vi "Input.vi"(8 "error in (no error)":errorcluster, 11 "Pump Calibration Config in":T1={"Settings"={"Cycle Period"=500.0, "Ismatech"={"VISA resource name"="", "Simulated?"=TRUE, "Pump Number"=1.0, "Reverse?"=FALSE}, "Masterflex"={"VISA resource name"="", "Simulated?"=TRUE, "Pump Number"=1.0, "Reverse?"=FALSE}, "Bronkhorst M13 Settings"={"VISA resource name"="", "Simulated?"=TRUE, "Smoothing Steps"=1}, "PID 2 Parameters"={"Input Device"=enum."Default", "Output Device"=enum."Default"}, "Tacmina Settings"={"Analog DAQ Task"="", "Digital DAQ Task"=""}, "KNF SIMDOS Settings"={"VISA resource name"="", "Simulated?"=TRUE}, "VICI M50 Settings"={"VISA resource name"="", "Pump ID"="", "Pump Head Vol"=0.0, "Reverse?"=FALSE, "Simulated?"=TRUE}, "FLOM Settings"={"VISA resource name"="", "Simulated?"=TRUE, "Pump Number"=0.0}, "Calibration Limits"={"Minimum (ml/min)"=0.0, "Maximum (ml/min)"=0.0, "Steps"=0.0}, "SSI PR Settings"={"VISA resource name"="", "Simulated?"=FALSE}, "Ismatech 4308 Settings"={"VISA resource name"="", "Pump Number"=1, "Channel Number"=0, "Simulated?"=TRUE, "Reverse?"=FALSE}, "Bronkhorst M14 Settings"={"VISA resource name"="", "Simulated?"=FALSE, "Smoothing Steps"=1}}, "Flowmeter Output"=0.0, "Density"=0.0, "FL Temp"=0.0, "Speed %"=0.0, "File Refnum"=refnum, "Pump On?"=enum."Not Initialized"} {"Settings"."Bronkhorst M14 Settings"."Smoothing Steps" min=1 step=1; "Settings"."Ismatech 4308 Settings"."Channel Number" min=0 max=3; "Settings"."Ismatech 4308 Settings"."Pump Number" min=1; "Settings"."Bronkhorst M13 Settings"."Smoothing Steps" min=1 step=1; "Settings"."Masterflex"."Pump Number" min=1.0 max=20.0 step=1.0; "Settings"."Ismatech"."Pump Number" min=1.0 max=20.0 step=1.0}) -> (0 "error out":errorcluster, 3 "Pump Calibration Config Out":T1={"Settings"={"Cycle Period"=500.0, "Ismatech"={"VISA resource name"="", "Simulated?"=TRUE, "Pump Number"=1.0, "Reverse?"=FALSE}, "Masterflex"={"VISA resource name"="", "Simulated?"=TRUE, "Pump Number"=1.0, "Reverse?"=FALSE}, "Bronkhorst M13 Settings"={"VISA resource name"="", "Simulated?"=TRUE, "Smoothing Steps"=1}, "PID 2 Parameters"={"Input Device"=enum."Default", "Output Device"=enum."Default"}, "Tacmina Settings"={"Analog DAQ Task"="", "Digital DAQ Task"=""}, "KNF SIMDOS Settings"={"VISA resource name"="", "Simulated?"=TRUE}, "VICI M50 Settings"={"VISA resource name"="", "Pump ID"="", "Pump Head Vol"=0.0, "Reverse?"=FALSE, "Simulated?"=TRUE}, "FLOM Settings"={"VISA resource name"="", "Simulated?"=TRUE, "Pump Number"=0.0}, "Calibration Limits"={"Minimum (ml/min)"=0.0, "Maximum (ml/min)"=0.0, "Steps"=0.0}, "SSI PR Settings"={"VISA resource name"="", "Simulated?"=FALSE}, "Ismatech 4308 Settings"={"VISA resource name"="", "Pump Number"=1, "Channel Number"=0, "Simulated?"=TRUE, "Reverse?"=FALSE}, "Bronkhorst M14 Settings"={"VISA resource name"="", "Simulated?"=FALSE, "Smoothing Steps"=1}}, "Flowmeter Output"=0.0, "Density"=0.0, "FL Temp"=0.0, "Speed %"=0.0, "File Refnum"=refnum, "Pump On?"=enum."Not Initialized"} {"Settings"."Bronkhorst M14 Settings"."Smoothing Steps" min=1 step=1; "Settings"."Ismatech 4308 Settings"."Channel Number" min=0 max=3; "Settings"."Ismatech 4308 Settings"."Pump Number" min=1; "Settings"."Bronkhorst M13 Settings"."Smoothing Steps" min=1 step=1; "Settings"."Masterflex"."Pump Number" min=1.0 max=20.0 step=1.0; "Settings"."Ismatech"."Pump Number" min=1.0 max=20.0 step=1.0})   [LabVIEW 2018, in "Calibration.lvlib" / "Engine.lvlib"]
uses:
  Engine.lvlib
  Pump Calibration Config.ctl
  Pfizer Timed Seq/Software/Ismatec ISM 831C/Controls/Ismatech ISM831C Settings Cluster.ctl
  Pfizer Timed Seq/Software/Masterflex 7550-30/Controls/Settings Cluster.ctl
  Pfizer Timed Seq/Software/Bronkhorst M13 Flow Meter/Settings Cluster.ctl
  Pfizer Timed Seq/Software/Measure Instrument/PID Input Enum.ctl
  Pfizer Timed Seq/Software/Measure Instrument/PID 2 Output Enum.ctl
  Pfizer Timed Seq/Software/Tacmina QI/Tacmina QI DAQ Setting.ctl
  Pfizer Timed Seq/Software/KNF Pump/Settings Cluster plus SIMDOS.ctl
  Pfizer Timed Seq/Software/VICI M50 Party Mode/Settings Cluster.ctl
  Pfizer Timed Seq/Software/FLOM Pump/Settings Cluster.ctl
  Pfizer Timed Seq/Software/SSI PR Class/SSI PR or LD Settings Cluster.ctl
  Pfizer Timed Seq/Software/Ismatec 78001/Ismatec 4083.ctl
  Pfizer Timed Seq/Software/Bronkhorst M14 Flow Meter/Settings Cluster.ctl
  Pfizer Timed Seq/Software/Bronkhorst M13 Flow Meter/Bronkhorst M13 Flow Meter.lvlib
  Pfizer Timed Seq/Software/Bronkhorst M14 Flow Meter/Bronkhorst M14 Flow Meter.lvlib
  Pfizer Timed Seq/Software/VICI M50 Party Mode/VICI M6 M50 Party Mode.lvlib
  Pfizer Timed Seq/Software/Ismatec ISM 831C/Ismatec ISM 831C.lvlib
  Pfizer Timed Seq/Software/Masterflex 7550-30/Masterflex 7550-30.lvlib
  Pfizer Timed Seq/Software/Tacmina QI/Tacmina QI.lvlib
  Pfizer Timed Seq/Software/KNF Pump/KNF SIMDOS.lvlib
  Pfizer Timed Seq/Software/FLOM Pump/FLOM Pump.lvlib
  Pfizer Timed Seq/Software/Calibration VIs/Calibration.lvlib
  Pfizer Timed Seq/Software/SSI PR Class/SSI PR or LD Pump.lvlib
  Pfizer Timed Seq/Software/Ismatec 78001/Ismatec 4308.lvlib
panel:
  # "Output Instruments"
  # "Input Instruments"
  # "Output Instruments"
  # "Input Instruments"
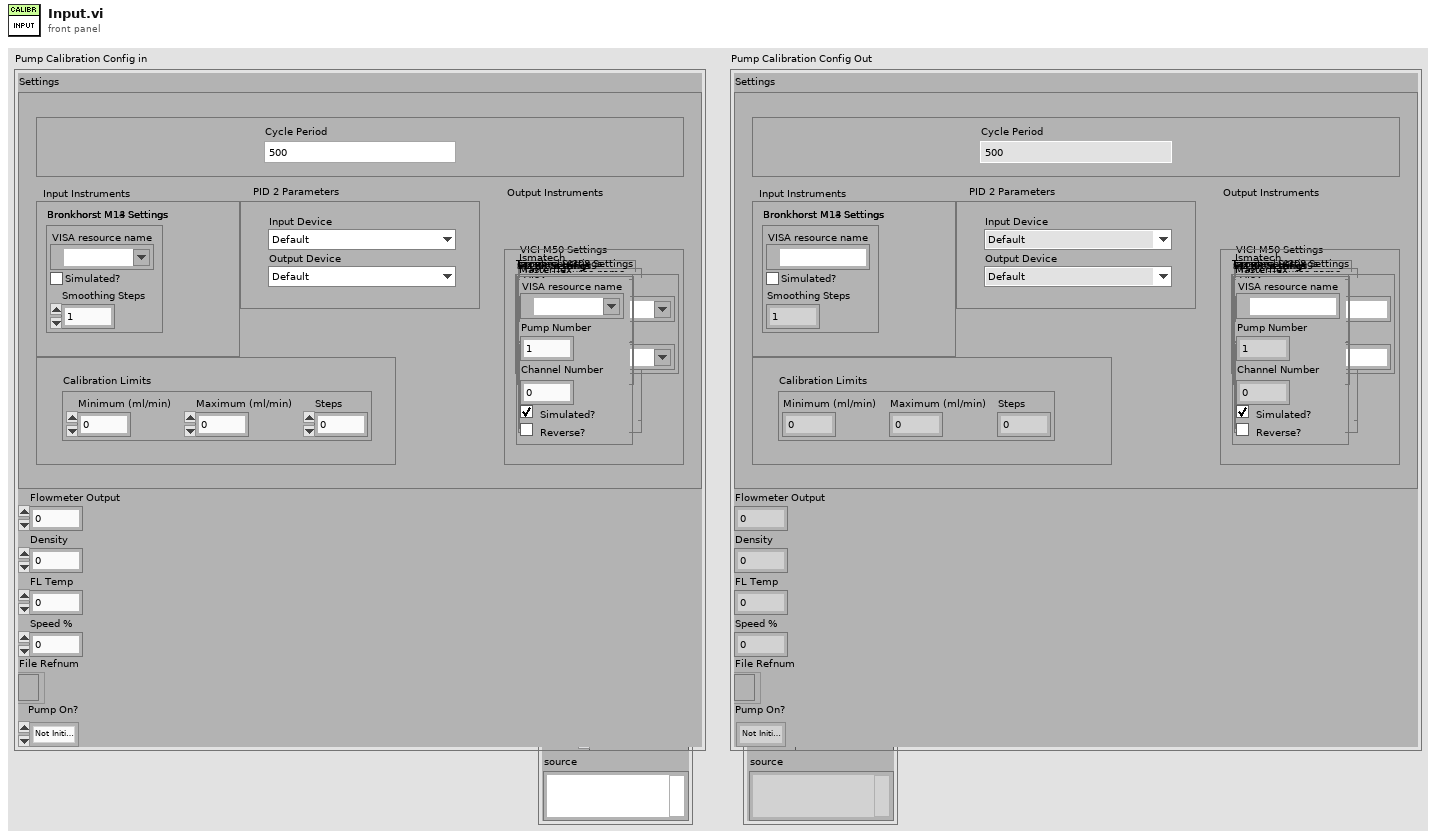
[diagram p1: front panel]
types:
  T1 = typedef "Calibration.lvlib/Pump Calibration Config.ctl" = cluster{"Settings":cluster{"Cycle Period":dbl, "Ismatech":T2, "Masterflex":T3, "Bronkhorst M13 Settings":T4, "PID 2 Parameters":cluster{"Input Device":T5, "Output Device":T6}, "Tacmina Settings":T7, "KNF SIMDOS Settings":T8, "VICI M50 Settings":T9, "FLOM Settings":T10, "Calibration Limits":cluster{"Minimum (ml/min)":dbl, "Maximum (ml/min)":dbl, "Steps":dbl}, "SSI PR Settings":T11, "Ismatech 4308 Settings":T12, "Bronkhorst M14 Settings":T13}, "Flowmeter Output":dbl, "Density":dbl, "FL Temp":dbl, "Speed %":dbl, "File Refnum":refnum<file>, "Pump On?":enum16{"Off", "On", "Not Initialized"}}
  T2 = typedef "Ismatec ISM 831C.lvlib/Ismatech ISM831C Settings Cluster.ctl" = cluster{"VISA resource name":refnum<visa-resource-name>, "Simulated?":bool, "Pump Number":dbl, "Reverse?":bool}
  T3 = typedef "Masterflex 7550-30.lvlib/Settings Cluster.ctl" = cluster{"VISA resource name":refnum<visa-resource-name>, "Simulated?":bool, "Pump Number":dbl, "Reverse?":bool}
  T4 = typedef "Bronkhorst M13 Flow Meter.lvlib/Settings Cluster.ctl" = cluster{"VISA resource name":refnum<visa-resource-name>, "Simulated?":bool, "Smoothing Steps":i32}
  T5 = typedef "PID Input Enum.ctl" = enum16{"Default", "Bronkhorst M13", "Bronkhorst M14", "Scale Rate of Change"}
  T6 = typedef "PID 2 Output Enum.ctl" = enum16{"Default", "Ismatec ISM 4308", "Ismatec ISM 831C", "Masterflex 7550-30", "VICI M6", "VICI M50", "Tacmina QI", "KNF SIMDOS", "ASIA Type C", "FLOM UI-22-11", "SSI PR/LD", "SSI P40", "Masterflex 75211-70"}
  T7 = typedef "Tacmina QI.lvlib/Tacmina QI DAQ Setting.ctl" = cluster{"Analog DAQ Task":refnum<k21>, "Digital DAQ Task":refnum<k21>}
  T8 = typedef "KNF SIMDOS.lvlib/Settings Cluster plus SIMDOS.ctl" = cluster{"VISA resource name":refnum<visa-resource-name>, "Simulated?":bool}
  T9 = typedef "VICI M6 M50 Party Mode.lvlib/Settings Cluster.ctl" = cluster{"VISA resource name":refnum<visa-resource-name>, "Pump ID":string, "Pump Head Vol":dbl, "Reverse?":bool, "Simulated?":bool}
  T10 = typedef "FLOM Pump.lvlib/Settings Cluster.ctl" = cluster{"VISA resource name":refnum<visa-resource-name>, "Simulated?":bool, "Pump Number":dbl}
  T11 = typedef "SSI PR or LD Pump.lvlib/SSI PR or LD Settings Cluster.ctl" = cluster{"VISA resource name":refnum<visa-resource-name>, "Simulated?":bool}
  T12 = typedef "Ismatec 4308.lvlib/Ismatec 4083.ctl" = cluster{"VISA resource name":refnum<visa-resource-name>, "Pump Number":i16, "Channel Number":i16, "Simulated?":bool, "Reverse?":bool}
  T13 = typedef "Bronkhorst M14 Flow Meter.lvlib/Settings Cluster.ctl" = cluster{"VISA resource name":refnum<visa-resource-name>, "Simulated?":bool, "Smoothing Steps":i32}
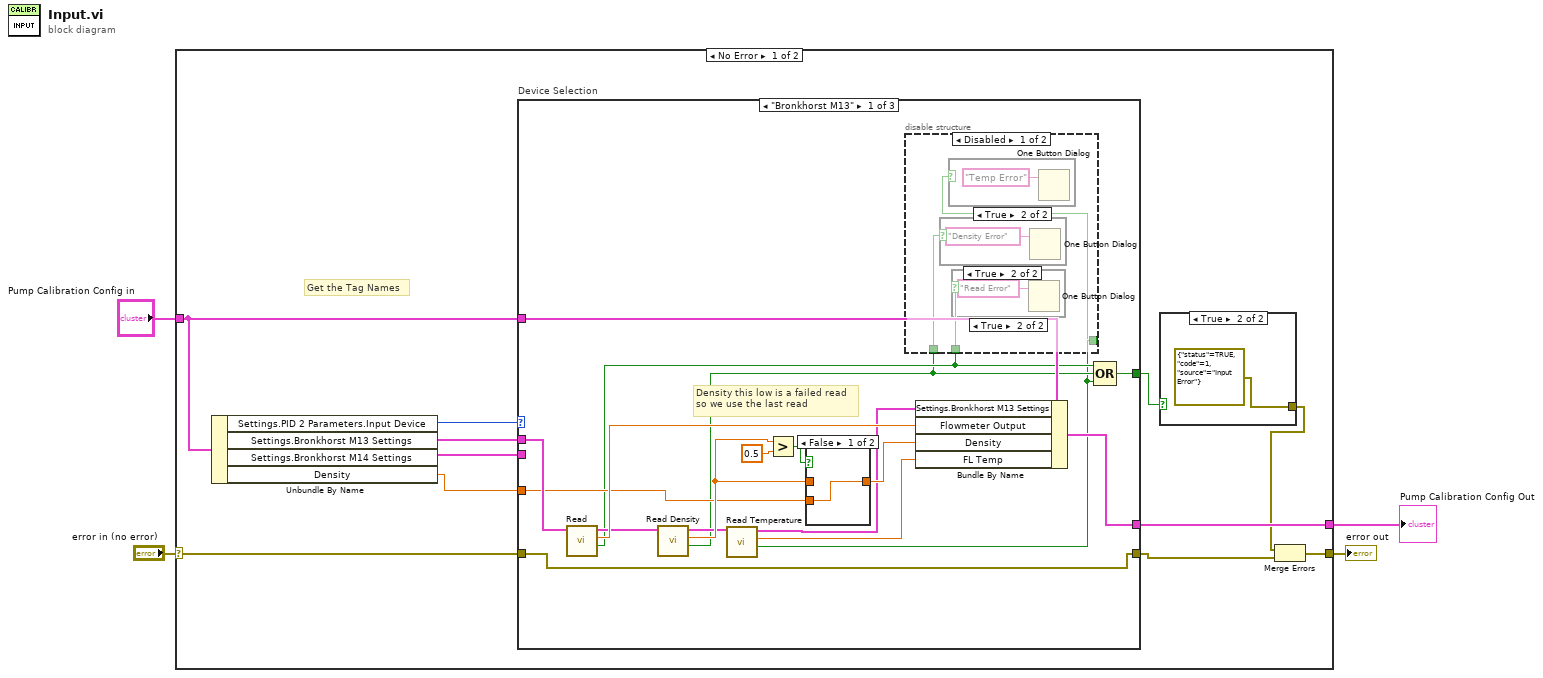
[diagram p0: block diagram]
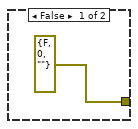
[diagram p2: hidden frame]
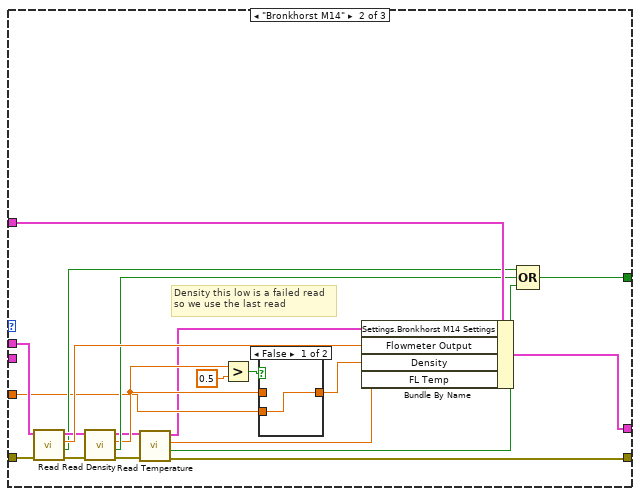
[diagram p8: hidden frame]
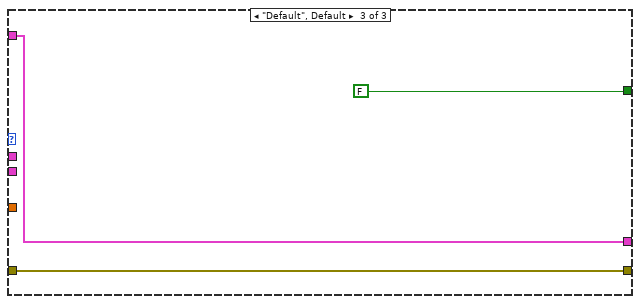
[diagram p10: hidden frame]
diagram:
  n1 = case shown="No Error" "error in (no error)" {
    selector: "error in (no error)" -> [w12 w71]
    tunnel: [w6 w71] -> w3
    tunnel: "Pump Calibration Config in" -> [w9 w70]
    tunnel: [w10 w70] -> w1
    frame No Error {
      # "Get the Tag Names"
      n2 = Unbundle By Name(w9) -> ("Settings.PID 2 Parameters.Input Device"=w15:T5, "Settings.Bronkhorst M13 Settings"=w14:T4, "Settings.Bronkhorst M14 Settings"=w13:T13, "Density"=w11:dbl)
      n3 = case "Device Selection" shown="\"Bronkhorst M13\"" w15 {
        tunnel: w9 -> [w35 w64 w69]
        tunnel: [w34 w63 w69] -> w10
        tunnel: w14 -> [w32 w60 _]
        tunnel: w13 -> [_ _ _]
        tunnel: w12 -> [w21 w61 w68]
        tunnel: [w21 w46 w68] -> w8
        tunnel: [w30 w55 FALSE ("Connection Error")] -> w5
        tunnel: w11 -> [w25 w50 _]
        frame "Bronkhorst M13" {
          # "Density this low is a failed read\nso we use the last read"
          n4 = call "Read.vi"("Bronkhorst Settings in"=w32) -> ("Connection Error"=w20:bool, "flow"=w33:dbl, "Bronkhorst Settings out"=w31:T4)  [unwired: 7 in, 1 out]
          n5 = call "Read Density.vi"("Bronkhorst Settings in"=w31) -> ("Connection Error"=w19:bool, "Density kg/m^3"=w27:sgl, "Bronkhorst Settings out"=w24:T4)  [unwired: 7 in, 1 out]
          n6 = call "Read Temperature.vi"("Bronkhorst Settings in"=w24) -> ("Connection Error"=w18:bool, "Temp (C)"=w22:sgl, "Bronkhorst Settings out"=w23:T4)  [unwired: 7 in, 1 out]
          n7 = Greater?(x=w27, y=sgl 0.5) -> (0:w29:bool)
          n8 = case shown="False" w29 {
            tunnel: w27 -> [_ w43]
            tunnel: [w42 w43] -> w26
            tunnel: w25 -> [w42 _]
            frame False {
            }
            frame True {
            }
          }
          n9 = disable-structure shown="Disabled" {
            disable-tunnel: w20 -> [w38 _]
            disable-tunnel: w19 -> [w37 _]
            disable-tunnel: w18 -> [w36 _]
            frame Disabled {
              n10 = case shown="True" w37 {
                frame False {
                }
                frame True {
                  n11 = One Button Dialog(message="Density Error") -> ()  [unwired: 1 in, 1 out]
                }
              }
              n12 = case shown="True" w36 {
                frame False {
                }
                frame True {
                  n13 = One Button Dialog(message="Temp Error") -> ()  [unwired: 1 in, 1 out]
                }
              }
              n14 = case shown="True" w38 {
                frame False {
                }
                frame True {
                  n15 = One Button Dialog(message="Read Error") -> ()  [unwired: 1 in, 1 out]
                }
              }
            }
            frame Enabled {
            }
          }
          n16 = Bundle By Name(cluster=w35, "Settings.Bronkhorst M13 Settings"=w23, "Flowmeter Output"=w33, "Density"=w26, "FL Temp"=w22) -> (w34:T1)
          n17 = Compound Arithmetic op=OR(w20, w19, w18) -> (w30:bool)
        }
        frame "Bronkhorst M14" {
          # "Density this low is a failed read\nso we use the last read"
          n18 = call "Read.vi"("error in (no error)"=w61, "Bronkhorst Settings in"=w60) -> ("error out"=w59:errorcluster, "Connection Error"=w57:bool, "flow"=w62:dbl, "Bronkhorst Settings out"=w58:T13)  [unwired: 6 in]
          n19 = call "Read Density.vi"("error in (no error)"=w59, "Bronkhorst Settings in"=w58) -> ("error out"=w49:errorcluster, "Connection Error"=w56:bool, "Density kg/m^3"=w52:sgl, "Bronkhorst Settings out"=w48:T4)  [unwired: 6 in]
          n20 = call "Read Temperature.vi"("error in (no error)"=w49, "Bronkhorst Settings in"=w48) -> ("error out"=w46:errorcluster, "Connection Error"=w44:bool, "Temp (C)"=w45:sgl, "Bronkhorst Settings out"=w47:T4)  [unwired: 6 in]
          n21 = Greater?(x=w52, y=sgl 0.5) -> (0:w54:bool)
          n22 = case shown="False" w54 {
            tunnel: w52 -> [_ w66]
            tunnel: [w65 w66] -> w51
            tunnel: w50 -> [w65 _]
            frame False {
            }
            frame True {
            }
          }
          n23 = Bundle By Name(cluster=w64, "Settings.Bronkhorst M14 Settings"=w47, "Flowmeter Output"=w62, "Density"=w51, "FL Temp"=w45) -> (w63:T1)
          n24 = Compound Arithmetic op=OR(w57, w56, w44) -> (w55:bool)
        }
        frame "Default", Default {
        }
      }
      n25 = case shown="True" w5 {
        tunnel: [errorcluster {"status"=FALSE, "code"=0, "source"=""} ("error constant") errorcluster {"status"=TRUE, "code"=1, "source"="Input Error"} ("error constant")] -> w7
        frame False {
        }
        frame True {
        }
      }
      n26 = Merge Errors(w7, w8) -> (w6:errorcluster)
    }
    frame Error {
    }
  }
  "error out" <- w3
  "Pump Calibration Config Out" <- w1
